vi "Allowed Terminal Modes.vi"(11 "Type Descriptor":T2) -> (1 "Single Mode String":string, 2 "Single Mode?":bool, 3 "Available Items":bool[](array[boolean]))   [LabVIEW 2020, in "Value Editor Base.lvclass"]
uses:
  Value Editor Base.lvclass
  Type Descriptor.ctl
  Terminal Direction.ctl
  Value Mode.ctl
  Special Terminal.ctl
  Terminal Mode.ctl
  Value Editor Base.lvclass/Value Editor Base.ctl
  FlexBlocks.lvlib
panel:
  in  "Terminal Mode (for properties)":T1
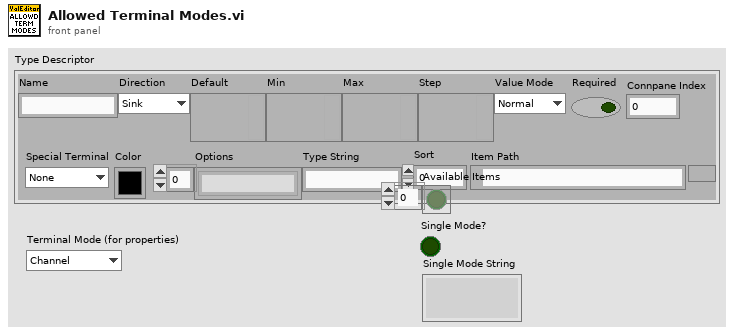
[diagram p1: front panel]
types:
  T1 = typedef "FlexBlocks.lvlib/Terminal Mode.ctl" = enum16{"Channel", "Config", "Value", "Control Ref"}
  T2 = typedef "FlexBlocks.lvlib/Type Descriptor.ctl" = cluster{"Name":string, "Direction":T3, "Default":variant, "Min":variant, "Max":variant, "Step":variant, "Value Mode":T4, "Required":bool, "Connpane Index":i32, "Special Terminal":T5, "Color":u32, "Options":string[], "Type String":string, "Sort":i32, "Item Path":path}
  T3 = typedef "FlexBlocks.lvlib/Terminal Direction.ctl" = enum16{"Sink", "Source"}
  T4 = typedef "FlexBlocks.lvlib/Value Mode.ctl" = enum16{"Normal", "Range", "Select"}
  T5 = typedef "FlexBlocks.lvlib/Special Terminal.ctl" = enum16{"None", "Action", "Init", "Tag", "State in", "State out", "Error"}
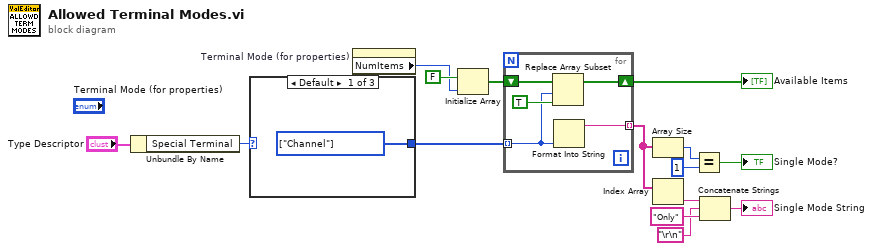
[diagram p0: block diagram]
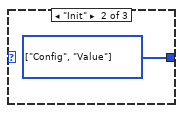
[diagram p2: hidden frame]
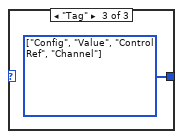
[diagram p3: hidden frame]
diagram:
  n1 = Unbundle By Name("Type Descriptor") -> ("Special Terminal"=w13:T5)
  n2 = case shown="Default" w13 {
    tunnel: [w16 w17 w18] -> w14
    frame Default {
      w16 = T1[] [enum."Channel"] items=["Channel", "Config", "Value", "Control Ref"] ("Array")
    }
    frame "Init" {
      w17 = T1[] [enum."Config", enum."Value"] items=["Channel", "Config", "Value", "Control Ref"] ("Array")
    }
    frame "Tag" {
      w18 = T1[] [enum."Config", enum."Value", enum."Control Ref", enum."Channel"] items=["Channel", "Config", "Value", "Control Ref"] ("Array")
    }
  }
  n3 = property on="Terminal Mode (for properties)" class="Enum (strict)"() -> ("NumItems"=w3:u32)  [unwired: 2 in, 2 out]
  n4 = Initialize Array(FALSE, w3) -> (w2:bool[])
  n5 = for {
    tunnel: w14 -> [w20] mode=indexing
    tunnel: [w23] -> w9 mode=indexing
    shift-right: [w19] -> w1
    shift-left: w2 -> [w22]
    n6 = Replace Array Subset(array=w22, new element=TRUE ("new element/subarray"), index=w20) -> (w19:bool[])
    n7 = Format Into String(w20) -> (resulting string=w23:string)  [unwired: 3 in, 1 out]
  }
  "Available Items" <- w1
  n8 = Array Size(array=w9) -> (size(s)=w12:i32)
  n9 = Index Array(array=w9) -> (element=w8:string)  [unwired: 1 in]
  n10 = Equal?(x=w12, y=1) -> (x = y?=→"Single Mode?":bool)
  n11 = Concatenate Strings(w8, "\r\n", "Only" ("string")) -> (→"Single Mode String":string)
